vi "反控启动.vi"(10 "启动参数":T1(ring)=enum."CODCr", 11 "启动类型":T2(ring)) -> ()   [LabVIEW 2016, in "MB SLAVE.lvlib"]
uses:
  MB SLAVE.lvlib
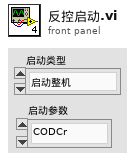
[diagram p1: front panel]
types:
  T1 = enum16{"未选择", "CODMn", "氨氮", "总磷", "总氮", "CODCr"}
  T2 = enum16{"启动整机", "停止整机", "标样核查", "加标回收", "平行样测试", "零点核查", "跨度核查", "校零", "校标"}
  T3 = enum16{"启动测量", "标样核查", "零点核查", "跨度核查", "空白测试", "平行样测试", "加标回收", "空白校准", "标样校准", "初始化（清洗）", "停止测试", "仪器重启", "校时", "模式设置", "测量间隔设置"}
  T4 = cluster{"测量模式":enum16{"水样测量", "标样核查", "零点核查", "跨度核查", "空白测试", "加标回收", "平行样", "校零", "校标"}}
  T5 = cluster{"status":bool, "代码":u16, "source":string}
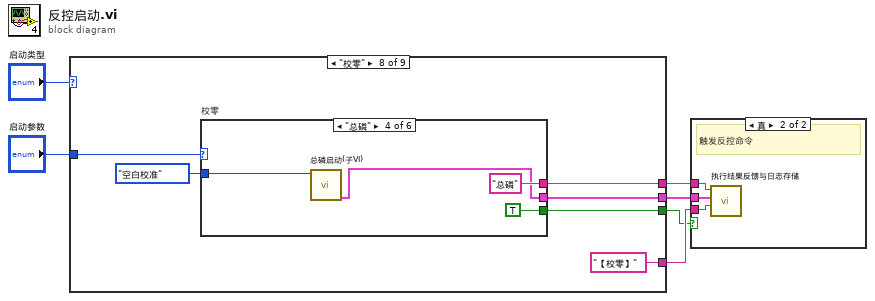
[diagram p0: block diagram]
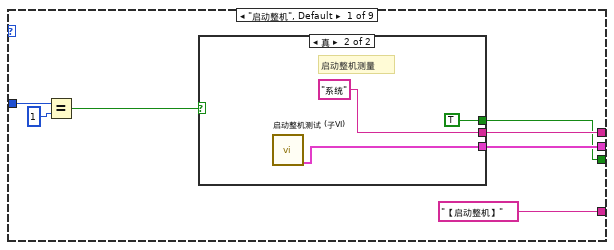
[diagram p3: hidden frame]
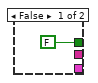
[diagram p4: hidden frame]
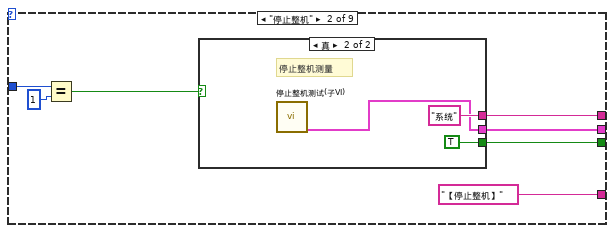
[diagram p5: hidden frame]
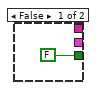
[diagram p6: hidden frame]
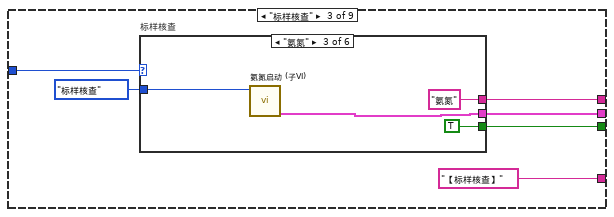
[diagram p7: hidden frame]
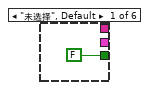
[diagram p8: hidden frame]
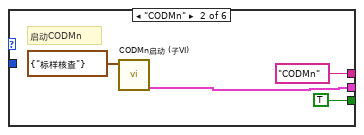
[diagram p9: hidden frame]
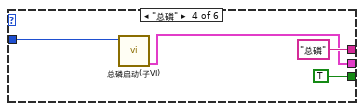
[diagram p10: hidden frame]
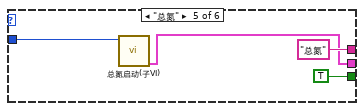
[diagram p11: hidden frame]
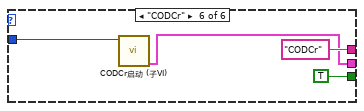
[diagram p12: hidden frame]
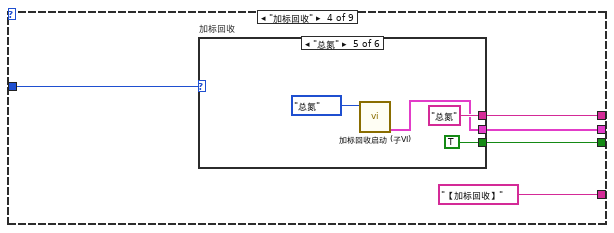
[diagram p13: hidden frame]
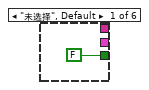
[diagram p14: hidden frame]
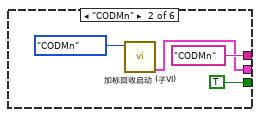
[diagram p15: hidden frame]
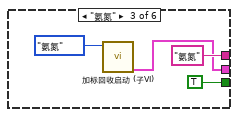
[diagram p16: hidden frame]
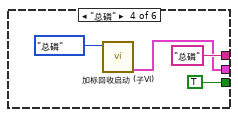
[diagram p17: hidden frame]
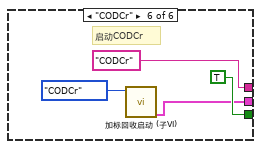
[diagram p18: hidden frame]
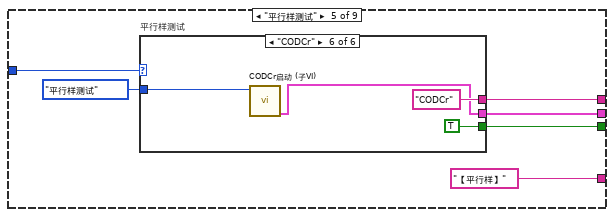
[diagram p19: hidden frame]
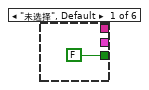
[diagram p20: hidden frame]
diagram:
  n1 = case shown="\"校零\"" "启动类型" {
    tunnel: "启动参数" -> [w13 w23 w34 w59 w87 w114 w141 w167 w194]
    tunnel: ["【启动整机】" ("日志信息") "【停止整机】" ("日志信息") "【标样核查】" ("日志信息") "【加标回收】" ("日志信息") "【平行样】" ("日志信息") "【零点核查】" ("日志信息") "【跨度核查】" ("日志信息") "【校零】" ("日志信息") "【校标】" ("日志信息")] -> w4
    tunnel: [w7 w19 w32 w57 w85 w111 w139 w165 w191] -> w3
    tunnel: [w10 w18 w31 w56 w84 w112 w138 w164 w192] -> w2
    tunnel: [w8 w20 w33 w58 w83 w110 w140 w166 w190] -> w1
    frame "启动整机", Default {
      n2 = Equal?(x=w13, y=1) -> (x = y?=w11:bool)
      n3 = case shown="真" w11 {
        tunnel: [_ w17] -> w10
        tunnel: [_ "系统" ("设备")] -> w8
        tunnel: [FALSE TRUE] -> w7
        frame False {
        }
        frame True {
          # "启动整机测量"
          n4 = call "启动整机测试 (子VI).vi"() -> ("error out"=w17:T5)  [unwired: 11 in]
        }
      }
    }
    frame "停止整机" {
      n5 = Equal?(x=w23, y=1) -> (x = y?=w22:bool)
      n6 = case shown="真" w22 {
        tunnel: [_ "系统" ("设备")] -> w20
        tunnel: [FALSE TRUE] -> w19
        tunnel: [_ w26] -> w18
        frame False {
        }
        frame True {
          # "停止整机测量"
          n7 = call "停止整机测试(子VI).vi"() -> ("error out"=w26:T5)  [unwired: 11 in]
        }
      }
    }
    frame "标样核查" {
      n8 = case "标样核查" shown="\"氨氮\"" w34 {
        tunnel: [_ "CODMn" ("设备") "氨氮" ("设备") "总磷" ("设备") "总氮" ("设备") "CODCr" ("设备")] -> w33
        tunnel: [_ w38 w43 w46 w50 w54] -> w31
        tunnel: [FALSE TRUE TRUE TRUE TRUE TRUE] -> w32
        tunnel: T3."标样核查" ("元素") -> [_ _ w40 w44 w48 w52]
        frame "未选择", Default {
        }
        frame "CODMn" {
          # "启动CODMn"
          n9 = call "CODMn启动 (子VI).vi"("启动测量模式"=T4 {"测量模式"=enum."标样核查"}) -> ("error out"=w38:T5)  [unwired: 10 in]
        }
        frame "氨氮" {
          n10 = call "氨氮启动 (子VI).vi"("元素"=w40) -> ("error out"=w43:T5)  [unwired: 10 in]
        }
        frame "总磷" {
          n11 = call "总磷启动(子VI).vi"("元素"=w44) -> ("error out"=w46:T5)  [unwired: 10 in]
        }
        frame "总氮" {
          n12 = call "总氮启动(子VI).vi"("元素"=w48) -> ("error out"=w50:T5)  [unwired: 10 in]
        }
        frame "CODCr" {
          n13 = call "CODCr启动 (子VI).vi"("元素"=w52) -> ("error out"=w54:T5)  [unwired: 10 in]
        }
      }
    }
    frame "加标回收" {
      n14 = case "加标回收" shown="\"总氮\"" w59 {
        tunnel: [_ "CODMn" ("设备") "氨氮" ("设备") "总磷" ("设备") "总氮" ("设备") "CODCr" ("设备")] -> w58
        tunnel: [_ w62 w66 w70 w74 w78] -> w56
        tunnel: [FALSE TRUE TRUE TRUE TRUE TRUE] -> w57
        frame "未选择", Default {
        }
        frame "CODMn" {
          n15 = call "加标回收启动 (子VI).vi"("启动参数"=T1."CODMn") -> ("error out"=w62:T5)  [unwired: 10 in]
        }
        frame "氨氮" {
          n16 = call "加标回收启动 (子VI).vi"("启动参数"=T1."氨氮") -> ("error out"=w66:T5)  [unwired: 10 in]
        }
        frame "总磷" {
          n17 = call "加标回收启动 (子VI).vi"("启动参数"=T1."总磷") -> ("error out"=w70:T5)  [unwired: 10 in]
        }
        frame "总氮" {
          n18 = call "加标回收启动 (子VI).vi"("启动参数"=T1."总氮") -> ("error out"=w74:T5)  [unwired: 10 in]
        }
        frame "CODCr" {
          # "启动CODCr"
          n19 = call "加标回收启动 (子VI).vi"("启动参数"=T1."CODCr") -> ("error out"=w78:T5)  [unwired: 10 in]
        }
      }
    }
    frame "平行样测试" {
      n20 = case "平行样测试" shown="\"CODCr\"" w87 {
        tunnel: [_ "CODMn" ("设备") "氨氮" ("设备") "总磷" ("设备") "总氮" ("设备") "CODCr" ("设备")] -> w83
        tunnel: [_ w91 w96 w99 w103 w107] -> w84
        tunnel: [FALSE TRUE TRUE TRUE TRUE TRUE] -> w85
        tunnel: T3."平行样测试" ("元素") -> [_ _ w93 w97 w101 w105]
        frame "未选择", Default {
        }
        frame "CODMn" {
          # "启动CODMn"
          n21 = call "CODMn启动 (子VI).vi"("启动测量模式"=T4 {"测量模式"=enum."平行样"}) -> ("error out"=w91:T5)  [unwired: 10 in]
        }
        frame "氨氮" {
          n22 = call "氨氮启动 (子VI).vi"("元素"=w93) -> ("error out"=w96:T5)  [unwired: 10 in]
        }
        frame "总磷" {
          n23 = call "总磷启动(子VI).vi"("元素"=w97) -> ("error out"=w99:T5)  [unwired: 10 in]
        }
        frame "总氮" {
          n24 = call "总氮启动(子VI).vi"("元素"=w101) -> ("error out"=w103:T5)  [unwired: 10 in]
        }
        frame "CODCr" {
          n25 = call "CODCr启动 (子VI).vi"("元素"=w105) -> ("error out"=w107:T5)  [unwired: 10 in]
        }
      }
    }
    frame "零点核查" {
      n26 = case "零点核查" shown="\"CODMn\"" w114 {
        tunnel: [_ "CODMn" ("设备") "氨氮" ("设备") "总磷" ("设备") "总氮" ("设备") "CODCr" ("设备")] -> w110
        tunnel: [_ w118 w123 w126 w130 w134] -> w112
        tunnel: [FALSE TRUE TRUE TRUE TRUE TRUE] -> w111
        tunnel: T3."零点核查" ("元素") -> [_ _ w120 w124 w128 w132]
        frame "未选择", Default {
        }
        frame "CODMn" {
          # "启动CODMn"
          n27 = call "CODMn启动 (子VI).vi"("启动测量模式"=T4 {"测量模式"=enum."零点核查"}) -> ("error out"=w118:T5)  [unwired: 10 in]
        }
        frame "氨氮" {
          n28 = call "氨氮启动 (子VI).vi"("元素"=w120) -> ("error out"=w123:T5)  [unwired: 10 in]
        }
        frame "总磷" {
          n29 = call "总磷启动(子VI).vi"("元素"=w124) -> ("error out"=w126:T5)  [unwired: 10 in]
        }
        frame "总氮" {
          n30 = call "总氮启动(子VI).vi"("元素"=w128) -> ("error out"=w130:T5)  [unwired: 10 in]
        }
        frame "CODCr" {
          # "启动CODCr"
          n31 = call "CODCr启动 (子VI).vi"("元素"=w132) -> ("error out"=w134:T5)  [unwired: 10 in]
        }
      }
    }
    frame "跨度核查" {
      n32 = case "跨度核查" shown="\"总磷\"" w141 {
        tunnel: [_ "CODMn" ("设备") "氨氮" ("设备") "总磷" ("设备") "总氮" ("设备") "CODCr" ("设备")] -> w140
        tunnel: [_ w145 w150 w153 w157 w161] -> w138
        tunnel: [FALSE TRUE TRUE TRUE TRUE TRUE] -> w139
        tunnel: T3."跨度核查" ("元素") -> [_ _ w147 w151 w155 w159]
        frame "未选择", Default {
        }
        frame "CODMn" {
          # "启动CODMn"
          n33 = call "CODMn启动 (子VI).vi"("启动测量模式"=T4 {"测量模式"=enum."跨度核查"}) -> ("error out"=w145:T5)  [unwired: 10 in]
        }
        frame "氨氮" {
          n34 = call "氨氮启动 (子VI).vi"("元素"=w147) -> ("error out"=w150:T5)  [unwired: 10 in]
        }
        frame "总磷" {
          n35 = call "总磷启动(子VI).vi"("元素"=w151) -> ("error out"=w153:T5)  [unwired: 10 in]
        }
        frame "总氮" {
          n36 = call "总氮启动(子VI).vi"("元素"=w155) -> ("error out"=w157:T5)  [unwired: 10 in]
        }
        frame "CODCr" {
          # "启动CODCr"
          n37 = call "CODCr启动 (子VI).vi"("元素"=w159) -> ("error out"=w161:T5)  [unwired: 10 in]
        }
      }
    }
    frame "校零" {
      n38 = case "校零" shown="\"总磷\"" w167 {
        tunnel: [_ "CODMn" ("设备") "氨氮" ("设备") "总磷" ("设备") "总氮" ("设备") "CODCr" ("设备")] -> w166
        tunnel: [_ w172 w177 w180 w184 w188] -> w164
        tunnel: [FALSE TRUE TRUE TRUE TRUE TRUE] -> w165
        tunnel: T3."空白校准" ("元素") -> [_ _ w174 w178 w182 w186]
        frame "未选择", Default {
        }
        frame "CODMn" {
          # "启动CODMn"
          n39 = call "CODMn启动 (子VI).vi"("启动测量模式"=T4 {"测量模式"=enum."校零"}) -> ("error out"=w172:T5)  [unwired: 10 in]
        }
        frame "氨氮" {
          n40 = call "氨氮启动 (子VI).vi"("元素"=w174) -> ("error out"=w177:T5)  [unwired: 10 in]
        }
        frame "总磷" {
          n41 = call "总磷启动(子VI).vi"("元素"=w178) -> ("error out"=w180:T5)  [unwired: 10 in]
        }
        frame "总氮" {
          n42 = call "总氮启动(子VI).vi"("元素"=w182) -> ("error out"=w184:T5)  [unwired: 10 in]
        }
        frame "CODCr" {
          # "启动CODCr"
          n43 = call "CODCr启动 (子VI).vi"("元素"=w186) -> ("error out"=w188:T5)  [unwired: 10 in]
        }
      }
    }
    frame "校标" {
      n44 = case "校标" shown="\"CODMn\"" w194 {
        tunnel: [_ "CODMn" ("设备") "氨氮" ("设备") "总磷" ("设备") "总氮" ("设备") "CODCr" ("设备")] -> w190
        tunnel: [_ w198 w203 w206 w210 w214] -> w192
        tunnel: [FALSE TRUE TRUE TRUE TRUE TRUE] -> w191
        frame "未选择", Default {
        }
        frame "CODMn" {
          # "启动CODMn"
          n45 = call "CODMn启动 (子VI).vi"("启动测量模式"=T4 {"测量模式"=enum."校标"}) -> ("error out"=w198:T5)  [unwired: 10 in]
        }
        frame "氨氮" {
          n46 = call "氨氮启动 (子VI).vi"("元素"=T3."标样校准") -> ("error out"=w203:T5)  [unwired: 10 in]
        }
        frame "总磷" {
          n47 = call "总磷启动(子VI).vi"("元素"=T3."标样校准") -> ("error out"=w206:T5)  [unwired: 10 in]
        }
        frame "总氮" {
          n48 = call "总氮启动(子VI).vi"("元素"=T3."标样校准") -> ("error out"=w210:T5)  [unwired: 10 in]
        }
        frame "CODCr" {
          n49 = call "CODCr启动 (子VI).vi"("元素"=T3."标样校准") -> ("error out"=w214:T5)  [unwired: 10 in]
        }
      }
    }
  }
  n50 = case shown="真" w3 {
    tunnel: w4 -> [_ w216]
    tunnel: w2 -> [_ w217]
    tunnel: w1 -> [_ w218]
    frame False {
    }
    frame True {
      # "触发反控命令"
      n51 = call "执行结果反馈与日志存储.vi"("日志信息"=w216, "error out"=w217, "设备"=w218) -> ()  [unwired: 9 in]
    }
  }
